vi "SECoP-simpleStringToJSON.vi"(11 "String in":string) -> (3 "String 3":string)   [LabVIEW 2015, in "SECoP.lvlib"]
uses:
  SECoP.lvlib
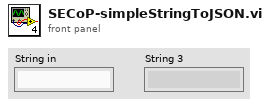
[diagram p1: front panel]
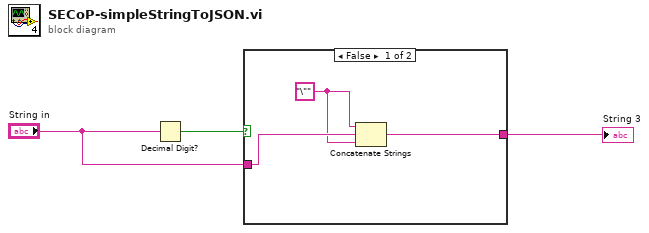
[diagram p0: block diagram]
diagram:
  n1 = Decimal Digit?(1:"String in") -> (0:w1:bool)
  n2 = case shown="False" w1 {
    tunnel: [w5 w7] -> w2
    tunnel: "String in" -> [w6 w7]
    frame False {
      w4 = "\""
      n3 = Concatenate Strings(w4, w6, w4) -> (w5:string)
    }
    frame True {
    }
  }
  "String 3" <- w2
